vi "WCA_SET_SIS_MODE.vi"(0 "Cartridge Band":u32=10, 1 "Slave Node in":cluster{"Address":i16, "Serial Number":i8[]}={"Address"=19, "Serial Number"=[16, 71, 55, 76, 1, 8, 0, -15]} {"Serial Number" format="%.0x"; "Address" format="%.0x"}, 2 "ObjHandle in":u32, 5 "POL":u32, 7 "sb":u32=1, 9 "SET_SIS_MODE":u8, 11 "error in (no error)":errorcluster) -> (4 "ObjHandle out":u32=92930112, 15 "error out":errorcluster)   [LabVIEW 2017]
uses:
  WCA_Global.vi
panel:
  # "Node Address"
  # "Serial Number"
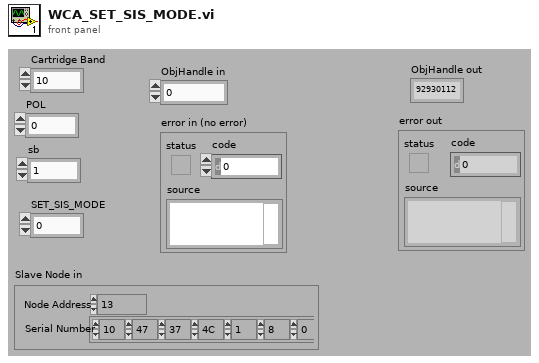
[diagram p1: front panel]
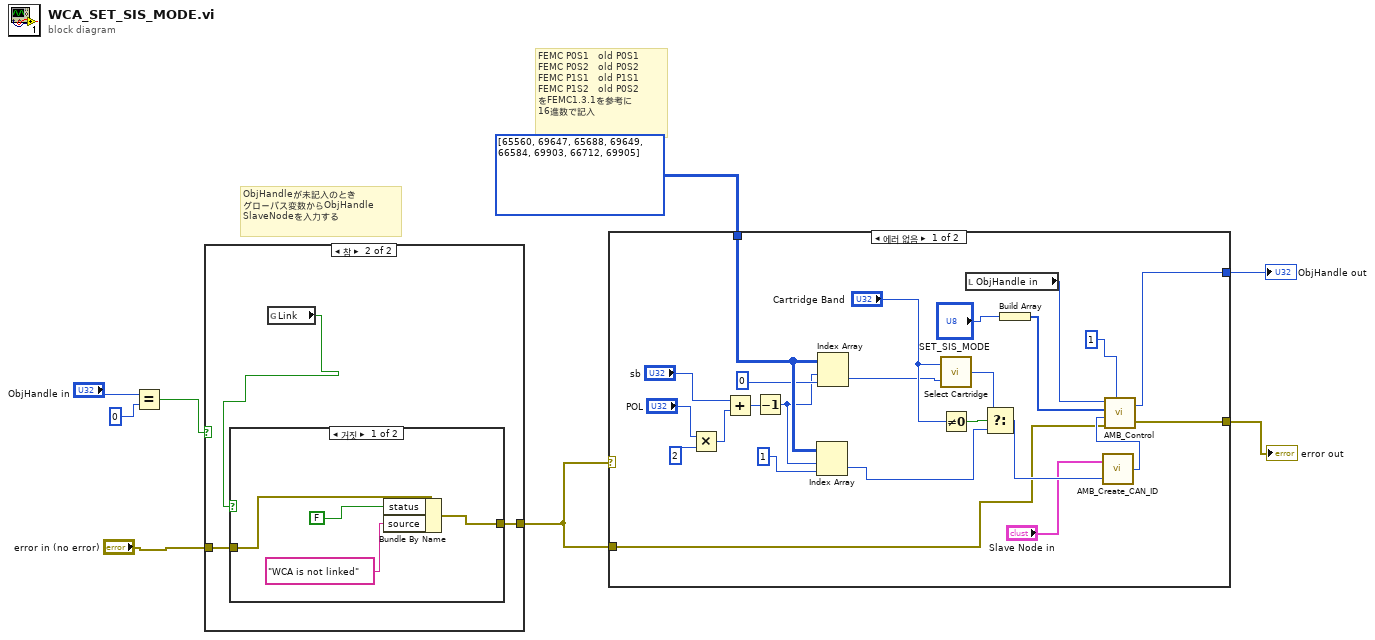
[diagram p0: block diagram]
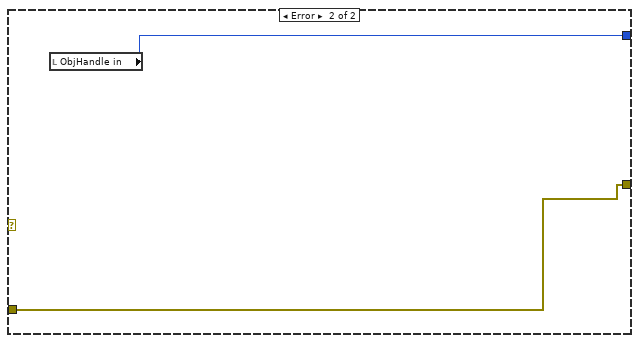
[diagram p2: hidden frame]
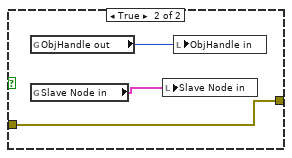
[diagram p4: hidden frame]
diagram:
  # "ObjHandleが未記入のとき\nグローバス変数からObjHandle\nSlaveNodeを入力する"
  # "FEMC P0S1   old P0S1\nFEMC P0S2   old P0S2\nFEMC P1S1   old P1S1\nFEMC P1S2   old P0S2\nをFEMC1.3.1を参考に\n16進数で記入"
  n1 = Equal?(x="ObjHandle in", y=0) -> (x = y?=w6:bool)
  n2 = case shown="참" w6 {
    tunnel: "error in (no error)" -> [w9 w12]
    tunnel: [w9 w11] -> w4
    frame False {
    }
    frame True {
      n3 = global read "WCA_Global.vi" "Link"() -> (w10:bool)
      n4 = case shown="거짓" w10 {
        tunnel: w12 -> [w16 w17]
        tunnel: [w13 w17] -> w11
        frame False {
          n5 = Bundle By Name(cluster=w16, "status"=FALSE, "source"="WCA is not linked") -> (w13:errorcluster)
        }
        frame True {
          n6 = global read "WCA_Global.vi" "ObjHandle out"() -> (w19:u32)
          n7 = global read "WCA_Global.vi" "Slave Node in"() -> (w18:cluster{"Address":i16, "Serial Number":i8[]})
          n8 = local write "Slave Node in"(w18) -> ()
          n9 = local write "ObjHandle in"(w19) -> ()
        }
      }
    }
  }
  n10 = case shown="에러 없음" w4 {
    tunnel: w4 -> [w37 w45]
    tunnel: [w35 w44] -> w3
    tunnel: [w34 w45] -> w2
    tunnel: i32[][] [[65560, 69647], [65688, 69649], [66584, 69903], [66712, 69905]] -> [w28 _]
    frame No Error {
      n11 = Multiply(x="POL", y=2) -> (x*y=w32:u32)
      n12 = Add(x="sb", y=w32) -> (x+y=w31:u32)
      n13 = Decrement(x=w31) -> (x-1=w24:u32)
      n14 = Index Array(array=w28, index (row)=w24, index (col)=1) -> (element=w29:i32)
      n15 = Index Array(array=w28, index (row)=w24, index (col)=0) -> (element=w30:i32)
      n16 = call "Select Cartridge.vi"("Relative Address in"=w30, "Cartridge band"="Cartridge Band") -> ("Relative Address out"=w41:u32)
      n17 = Not Equal To 0?(x="Cartridge Band") -> (x != 0?=w42:bool)
      n18 = local read "ObjHandle in"() -> (w36:u32)
      n19 = Select(t=w41, s=w42, f=w29) -> (s? t:f=w40:u32)
      n20 = Build Array("SET_SIS_MODE") -> (w20:u8[])
      n21 = call "AMB_Create_CAN_ID.vi"("Relative Address in"=w40, "Slave Node in"="Slave Node in") -> ("CAN ID out"=w43:u32)
      n22 = call "AMB_Control.vi"("ObjHandle in"=w36, "Data in"=w20, "CAN ID in"=w43, "error in"=w37, "Data Length in"=1) -> ("ObjHandle out"=w35:u32, "error out"=w34:errorcluster)
    }
    frame Error {
      n23 = local read "ObjHandle in"() -> (w44:u32)
    }
  }
  "ObjHandle out" <- w3
  "error out" <- w2
